vi "Config Alternate Amplitude.vi"(0 "VISA Resource Name":refnum<visa-resource-name>, 1 "State (F: OFF)":bool, 2 "Trigger Source  (0: Internal)":enum16{"Internal", "External", "Manual"}(ring) format="%.0g", 3 "Manual Trigger (0: Main)":enum16{"Main", "Delta"}(ring) format="%.0g", 4 "Amplitude (0.0)":dbl, 5 "error in (no error)":errorcluster {"code" format="%.0x"}) -> (14 "VISA Resource Name Out":refnum<visa-resource-name>, 19 "error out":errorcluster {"code" format="%.0x"})   [LabVIEW 2012, in "Agilent ESG Series.lvlib"]
doc: "This VI configures alternate amplitude.\n\nNotes:\n(1) This VI is supported for Agilent 44xxB with option UNA or Agilent E4438C only."
uses:
  <instrlib>/Agilent ESG Series/Agilent ESG Series.lvlib
panel:
  # "ON"
  # "OFF"
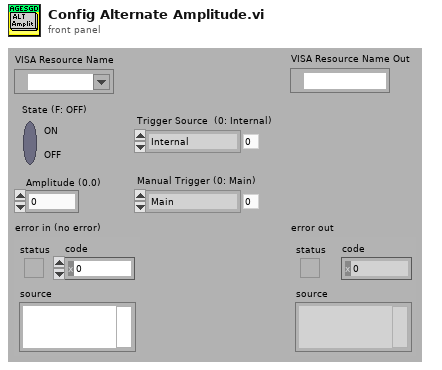
[diagram p1: front panel]
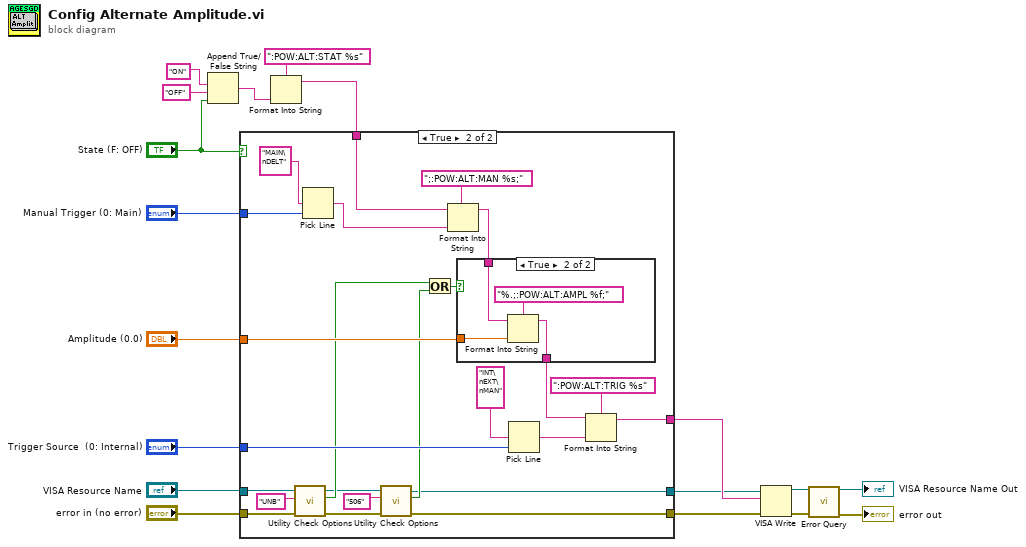
[diagram p0: block diagram]
diagram:
  n1 = Append True/False String(1:"State (F: OFF)", 2:"OFF" ("false string"), 3:"ON" ("multi-line string")) -> (0:w8:string)  [unwired: 1 in]
  n2 = Format Into String(format string=":POW:ALT:STAT %s", w8) -> (resulting string=w6:string)  [unwired: 2 in, 1 out]
  n3 = case shown="True" "State (F: OFF)" {
    tunnel: "Amplitude (0.0)" -> [_ w42]
    tunnel: "Manual Trigger (0: Main)" -> [_ w40]
    tunnel: "Trigger Source  (0: Internal)" -> [_ w36]
    tunnel: w6 -> [w21 w33]
    tunnel: [w21 w30] -> w5
    tunnel: "VISA Resource Name" -> [w20 w24]
    tunnel: [w20 w22] -> w3
    tunnel: "error in (no error)" -> [w19 w25]
    tunnel: [w19 w26] -> w1
    frame False {
    }
    frame True {
      n4 = call <instrlib>:"Utility Check Options.vi"("error in (no error)"=w25, "Search Options"="UNB", "VISA Resource Name"=w24) -> ("error out"=w27:errorcluster, "Found"=w29:bool, "VISA Resource Name Out"=w23:refnum<visa-resource-name>)  [unwired: 6 in]
      n5 = Pick Line(multi-line string="MAIN\nDELT", line index=w40) -> (output string=w38:string)  [unwired: 1 in]
      n6 = call <instrlib>:"Utility Check Options.vi"("error in (no error)"=w27, "Search Options"="506", "VISA Resource Name"=w23) -> ("error out"=w26:errorcluster, "Found"=w28:bool, "VISA Resource Name Out"=w22:refnum<visa-resource-name>)  [unwired: 6 in]
      n7 = Or(x=w29, y=w28) -> (x .or. y?=w43:bool)
      n8 = Format Into String(format string=";:POW:ALT:MAN %s;", initial string=w33, w38) -> (resulting string=w31:string)  [unwired: 1 in, 1 out]
      n9 = case shown="True" w43 {
        tunnel: w42 -> [_ w49]
        tunnel: [w46 w48] -> w32
        tunnel: w31 -> [w46 w47]
        frame False {
        }
        frame True {
          n10 = Format Into String(format string="%.;:POW:ALT:AMPL %f;", initial string=w47, w49) -> (resulting string=w48:string)  [unwired: 1 in, 1 out]
        }
      }
      n11 = Pick Line(multi-line string="INT\nEXT\nMAN", line index=w36) -> (output string=w34:string)  [unwired: 1 in]
      n12 = Format Into String(format string=":POW:ALT:TRIG %s", initial string=w32, w34) -> (resulting string=w30:string)  [unwired: 1 in, 1 out]
    }
  }
  n13 = VISA Write(VISA resource name=w3, write buffer=w5, error in (no error)=w1) -> (VISA resource name out=w16:refnum<visa-resource-name>, error out=w15:errorcluster)  [unwired: 1 out]
  n14 = call <instrlib>:"Error Query.vi"("VISA Resource Name"=w16, "error in (no error)"=w15) -> ("VISA Resource Name Out"=→"VISA Resource Name Out":refnum<visa-resource-name>, "error out"=→"error out":errorcluster)  [unwired: 10 in, 2 out]
